vi "CRYMake Phase Index.vi"(10 "Mag_Phase Flag":bool, 11 "Selected Rows In":i32[](array[numeric])) -> (2 "Mag_Phase":bool[](array[boolean]), 3 "Selected Rows Out":i32[](array[numeric]))   [LabVIEW 2013]
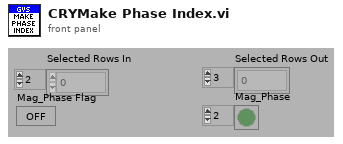
[diagram p1: front panel]
types:
  T1 = typedef "CRYData Cluster.ctl" = cluster{"Name":string, "Curve":cluster{"x":dbl, "y":dbl, "z":dbl}[], "X data":u16, "Y data":u16, "Z data":u16, "X axis":u16, "Y axis":u16, "Z axis":u16, "X unit":string, "Y unit":string, "Z unit":string, "X dB ref":dbl, "Y dB ref":dbl, "Z dB ref":dbl, "single val":bool, "protected":bool, "display X":bool, "display Y":bool, "display Z":bool, "Test Info":string, "Step No.":i32, "Plot Settings":cluster{"Color":u32, "Interpolation":u8, "Point Style":u8, "Line Style":u8, "Point Color":u32, "Line Width":u8, "Bar Plot Style":u8, "Fill To":i16}, "AutoProtect":bool}
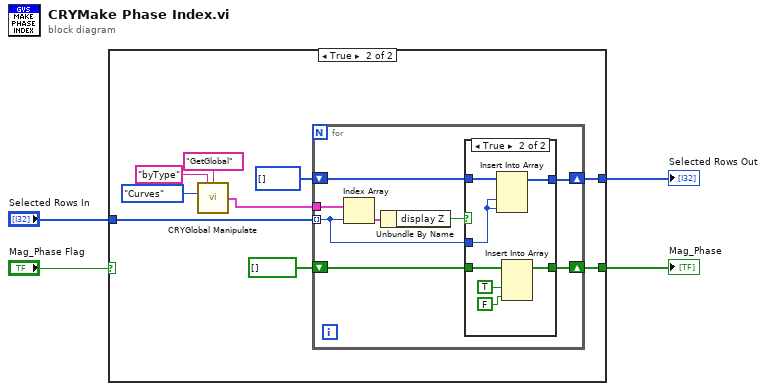
[diagram p0: block diagram]
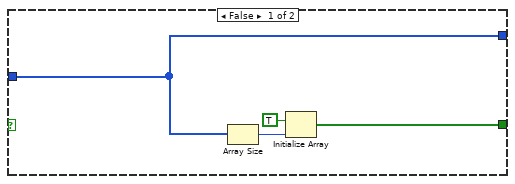
[diagram p2: hidden frame]
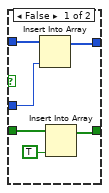
[diagram p3: hidden frame]
diagram:
  n1 = case shown="True" "Mag_Phase Flag" {
    tunnel: "Selected Rows In" -> [w6 w15]
    tunnel: [w6 w14] -> w3
    tunnel: [w5 w13] -> w2
    frame False {
      n2 = Array Size(array=w6) -> (size(s)=w8:i32)
      n3 = Initialize Array(TRUE ("x .and. y?"), w8) -> (w5:bool[])
    }
    frame True {
      n4 = call "CRYGlobal Manipulate.vi"("Type"=enum16{"Curves", "Values", "Results", "WFM"}."Curves", "sOption"="byType", "sAction"="GetGlobal") -> ("Curves Out"=w9:T1[])  [unwired: 6 in, 6 out]
      n5 = for {
        tunnel: w15 -> [w21] mode=indexing
        tunnel: w9 -> [w25]
        shift-right: [w22] -> w14
        shift-left: i32[] [] ("Selected Rows In") -> [w23]
        shift-right: [w19] -> w13
        shift-left: bool[] [] -> [w18]
        n6 = Index Array(array=w25, index=w21) -> (element=w24:T1)
        n7 = Unbundle By Name(w24) -> ("display Z"=w20:bool)
        n8 = case shown="True" w20 {
          tunnel: w23 -> [w31 w38]
          tunnel: [w30 w37] -> w22
          tunnel: w21 -> [w29 w36]
          tunnel: [w26 w33] -> w19
          tunnel: w18 -> [w27 w35]
          frame False {
            n9 = Insert Into Array(array=w31, new element=w29) -> (w30:i32[])  [unwired: 1 in]
            n10 = Insert Into Array(array=w27, new element=TRUE ("new element/subarray")) -> (w26:bool[])  [unwired: 1 in]
          }
          frame True {
            n11 = Insert Into Array(array=w38, new element #1=w36, new element #2=w36) -> (w37:i32[])  [unwired: 1 in]
            n12 = Insert Into Array(array=w35, new element #1=TRUE ("new element/subarray"), new element #2=FALSE ("new element/subarray")) -> (w33:bool[])  [unwired: 1 in]
          }
        }
      }
    }
  }
  "Selected Rows Out" <- w3
  "Mag_Phase" <- w2
